vi "DependencyFilter.vi"(9 "FilterOptions":T1, 11 "LibraryDependency In":map{path, T2}(c390)) -> (3 "Filtered LibraryDependency Out":map{path, T2}(c390))   [LabVIEW 2020, in "DependencyChecker.lvlib"]
uses:
  DependencyChecker.lvlib
  LibraryDependentInfo.vi
  <vilib>/Utility/lvfile.llb/FT_FileTypes.ctl
  FilterOptions.ctl
  <vilib>/Utility/lvfile.llb/NI_FileType.lvlib
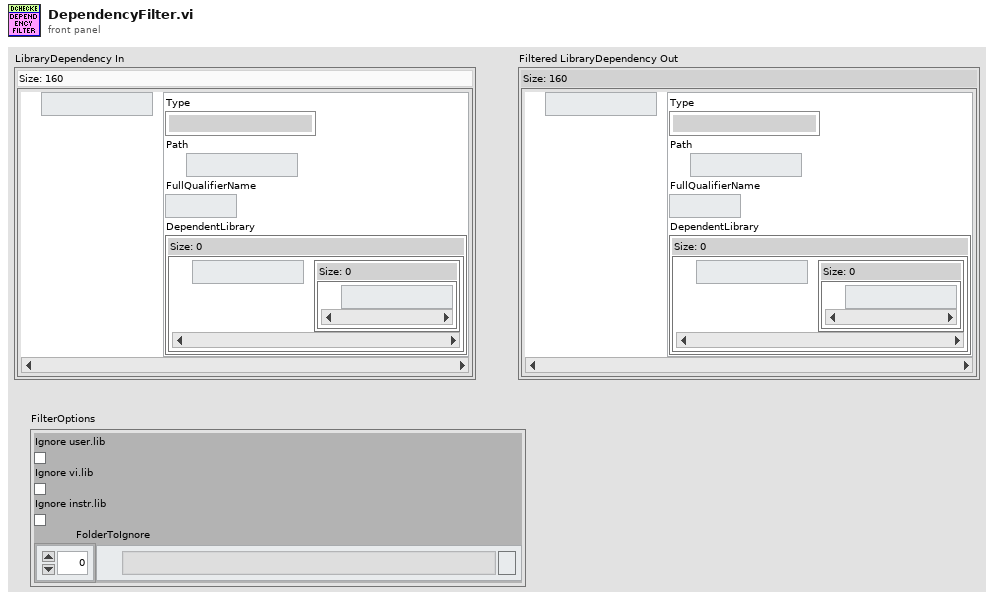
[diagram p1: front panel]
types:
  T1 = typedef "DependencyChecker.lvlib/FilterOptions.ctl" = cluster{"Ignore user.lib":bool, "Ignore vi.lib":bool, "Ignore instr.lib":bool, "FolderToIgnore":path[]}
  T2 = typedef "DependencyChecker.lvlib/LibraryDependentInfo.vi" = cluster{"Type":T3, "Path":path, "FullQualifierName":string, "DependentLibrary":map{path, set{path}}}
  T3 = typedef "NI_FileType.lvlib/FT_FileTypes.ctl" = enum32{"Invalid file/path", "Unknown type", "Instrument", "Control", "Polymorphic VI", "Project", "Library", "LVClass", "XControl", "XNode", "CIN", "Run-time menu", "Palette menu", "LLB", "Shortcut", "Directory", "Class Private Data Control", "Statechart", "MathScript .m file", "Ladder Diagram", "LVLibp"}
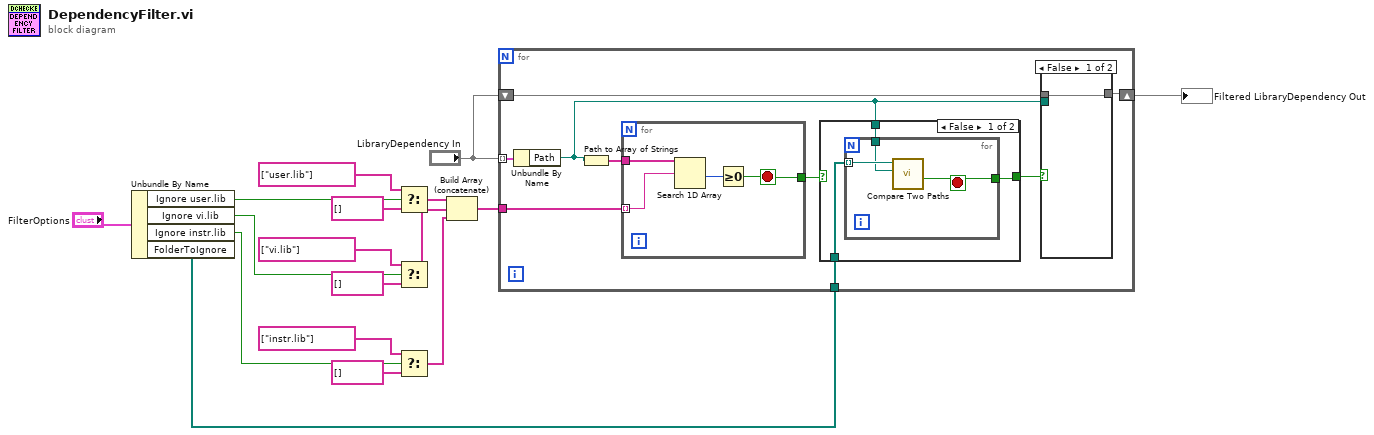
[diagram p0: block diagram]
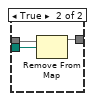
[diagram p3: hidden frame]
diagram:
  n1 = Unbundle By Name("FilterOptions") -> ("Ignore user.lib"=w15:bool, "Ignore vi.lib"=w8:bool, "Ignore instr.lib"=w7:bool, "FolderToIgnore"=w2:path[])
  n2 = Select(t=string[] ["user.lib"], s=w15, f=string[] []) -> (s? t:f=w6:string[])
  n3 = Select(t=string[] ["vi.lib"], s=w8, f=string[] []) -> (s? t:f=w5:string[])
  n4 = Select(t=string[] ["instr.lib"], s=w7, f=string[] []) -> (s? t:f=w4:string[])
  n5 = Build Array (concatenate)(w6, w5, w4) -> (w3:string[])
  n6 = for {
    tunnel: "LibraryDependency In" -> [w26] mode=indexing
    shift-right: [w22] -> w1
    shift-left: "LibraryDependency In" -> [w23]
    tunnel: w3 -> [w24]
    tunnel: w2 -> [w19]
    n7 = Unbundle By Name(w26) -> ("Path"=w18:path)
    n8 = Path to Array of Strings(0:w18) -> (2:w25:string[])  [unwired: 1 out]
    n9 = for {
      tunnel: w25 -> [w41]
      tunnel: w24 -> [w40] mode=indexing
      tunnel: [w38] -> w21
      stop <- w38 stop-if-true
      n10 = Search 1D Array(1D array=w41, element=w40) -> (index of element=w39:i32)  [unwired: 1 in]
      n11 = Greater Or Equal To 0?(x=w39) -> (x >= 0?=w38:bool)
    }
    n12 = case shown="False" w21 {
      selector: w21 -> [_ w33]
      tunnel: [w27 w33] -> w20
      tunnel: w19 -> [w29 _]
      tunnel: w18 -> [w28 _]
      frame False {
        n13 = for {
          tunnel: w29 -> [w32] mode=indexing
          tunnel: w28 -> [w31]
          tunnel: [w30] -> w27
          stop <- w30 stop-if-true
          n14 = call <vilib>:"Compare Two Paths.vi"("Path 2"=w31, "Path 1"=w32) -> ("Path 2 Relative to Path 1?"=w30:bool)  [unwired: 6 in, 3 out]
        }
      }
      frame True {
      }
    }
    n15 = case shown="False" w20 {
      tunnel: w23 -> [w34 w37]
      tunnel: w18 -> [_ w36]
      tunnel: [w34 w35] -> w22
      frame False {
      }
      frame True {
        n16 = Remove From Map(10:w36, 11:w37) -> (3:w35:map{path, T2})  [unwired: 2 out]
      }
    }
  }
  "Filtered LibraryDependency Out" <- w1
